vi "HandleEvent.vi"(4 "Queue In":refnum<queue>, 5 "Event Data":cluster{"sender":refnum<k24>, "e":refnum<k24>}, 6 "Control Ref":refnum<k24>, 7 "Event Universal Data":T1) -> ()   [LabVIEW 2017, in "LiteAgentSDK.lvlib"]
uses:
  LiteAgentSDK.lvlib
  C:/Users/Jan/Projects/LiteAgentSDK-LabVIEW/Source/Bin/LiteAgentSDK.LabVIEW.dll
  Bin/LiteAgentSDK.LabVIEW.dll
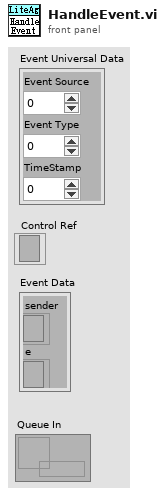
[diagram p1: front panel]
types:
  T1 = cluster{"Event Source":i32, "Event Type":u32, "TimeStamp":u32}
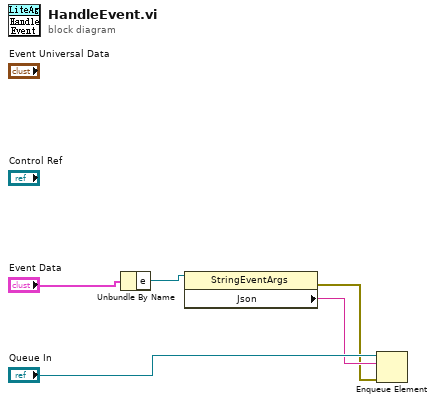
[diagram p0: block diagram]
diagram:
  n1 = Unbundle By Name("Event Data") -> ("e"=w3:refnum<k24>)
  n2 = property on="属性节点" class="StringEventArgs"(reference=w3) -> (error out=w1:errorcluster, "Json"=w2:string)  [unwired: 1 in, 1 out]
  n3 = Enqueue Element(queue="Queue In", element=w2, error in (no error)=w1) -> ()  [unwired: 1 in, 3 out]
